vi "AuMT8852B Dirty Parameter Table.vi"(0 "VISA session":refnum<visa-resource-name>, 1 "Test (Single-slot sensitivity)":T1(ring), 2 "Variable (Frequency offset)":T2(ring), 3 "Range check? (F)":bool, 4 "Simulate? (F)":bool, 5 "error in (no error)":errorcluster, 6 "Set/Get (Set)":enum16{"Set", "Get"}(ring), 8 "Script (3)":i32=3, 10 "Parameters":dbl[](array[numeric]) format="%.2f") -> (13 "Parameters out":dbl[](array[numeric]) format="%.2f", 14 "VISA session out":refnum<visa-resource-name>, 19 "error out":errorcluster)   [LabVIEW 2017]
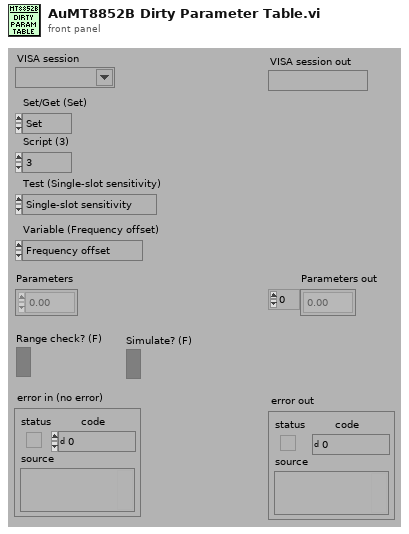
[diagram p1: front panel]
types:
  T1 = enum16{"Single-slot sensitivity", "Multiple-slot sensitivity", "EDR sensitivity"}
  T2 = enum16{"Frequency offset", "Symbol timing value", "Mod index value"}
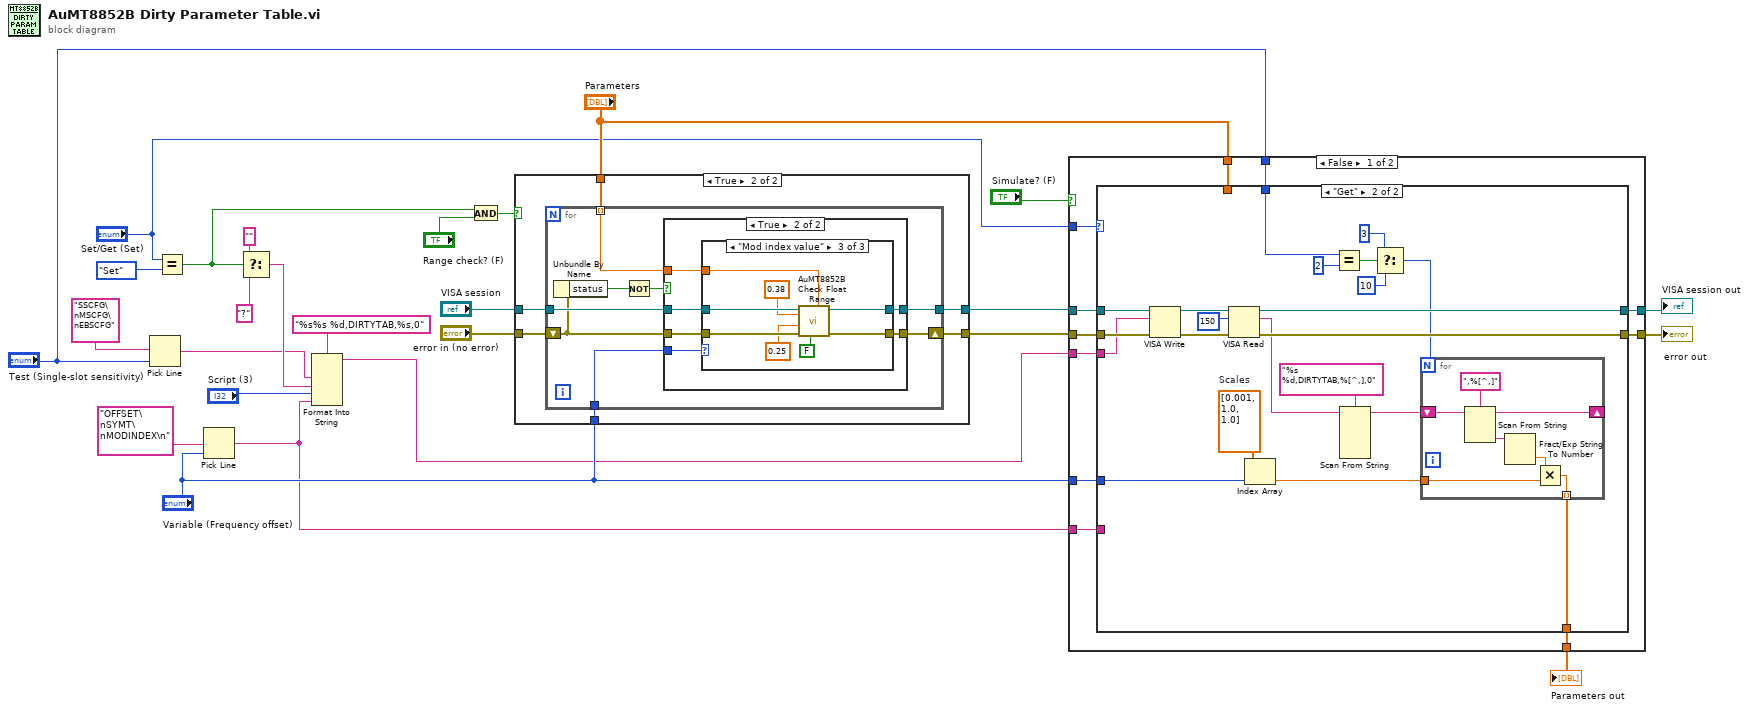
[diagram p0: block diagram]
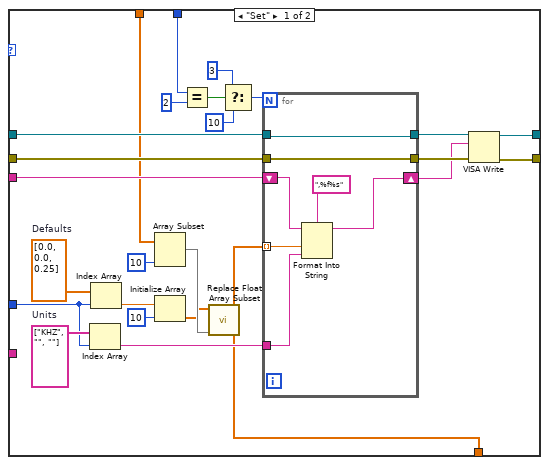
[diagram p2: hidden frame]
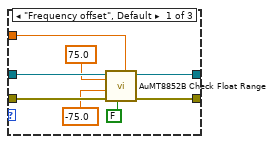
[diagram p6: hidden frame]
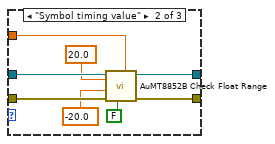
[diagram p7: hidden frame]
diagram:
  n1 = Pick Line(multi-line string="SSCFG\nMSCFG\nEBSCFG", line index="Test (Single-slot sensitivity)") -> (output string=w2:string)  [unwired: 1 in]
  n2 = Equal?(x="Set/Get (Set)", y=enum16{"Set", "Get"}."Set") -> (x = y?=w15:bool)
  n3 = Pick Line(multi-line string="OFFSET\nSYMT\nMODINDEX\n", line index="Variable (Frequency offset)") -> (output string=w5:string)  [unwired: 1 in]
  n4 = Select(t="", s=w15, f="?") -> (s? t:f=w21:string)
  n5 = Format Into String(format string="%s%s %d,DIRTYTAB,%s,0" ("Format String"), w2, w21, "Script (3)", w5) -> (resulting string=w6:string)  [unwired: 2 in, 1 out]
  n6 = And(x=w15, y="Range check? (F)") -> (x .and. y?=w17:bool)
  n7 = case shown="True" w17 {
    tunnel: "VISA session" -> [w28 w34]
    tunnel: "error in (no error)" -> [w27 w30]
    tunnel: [w28 w33] -> w13
    tunnel: [w27 w29] -> w14
    tunnel: "Parameters" -> [_ w32]
    tunnel: "Variable (Frequency offset)" -> [_ w31]
    frame False {
    }
    frame True {
      n8 = for {
        tunnel: w34 -> [w42]
        tunnel: [w41] -> w33
        tunnel: w32 -> [w39] mode=indexing
        tunnel: w31 -> [w40]
        shift-right: [w36] -> w29
        shift-left: w30 -> [w35]
        n9 = Unbundle By Name(w35) -> ("status"=w37:bool)
        n10 = Not(x=w37) -> (.not. x?=w38:bool)
        n11 = case shown="True" w38 {
          tunnel: w42 -> [w43 w50]
          tunnel: w35 -> [w44 w49]
          tunnel: [w43 w48] -> w41
          tunnel: [w44 w47] -> w36
          tunnel: w40 -> [_ w46]
          tunnel: w39 -> [_ w45]
          frame False {
          }
          frame True {
            n12 = case shown="\"Mod index value\"" w46 {
              tunnel: w50 -> [w58 w66 w74]
              tunnel: w49 -> [w57 w65 w73]
              tunnel: [w56 w64 w72] -> w48
              tunnel: [w55 w63 w71] -> w47
              tunnel: w45 -> [w51 w59 w67]
              frame "Frequency offset", Default {
                n13 = call <instrlib>:"AuMT8852B Check Float Range.vi"("Value (0)"=w51, "Check IVI flag first? (T)"=FALSE, "error in (no error)"=w57, "Lower limit (-1)"=-75.0, "Upper limit (1)"=75.0, "VISA session"=w58) -> ("error out"=w55:errorcluster, "VISA session out"=w56:refnum<visa-resource-name>)  [unwired: 4 in]
              }
              frame "Symbol timing value" {
                n14 = call <instrlib>:"AuMT8852B Check Float Range.vi"("Value (0)"=w59, "Check IVI flag first? (T)"=FALSE, "error in (no error)"=w65, "Lower limit (-1)"=-20.0, "Upper limit (1)"=20.0, "VISA session"=w66) -> ("error out"=w63:errorcluster, "VISA session out"=w64:refnum<visa-resource-name>)  [unwired: 4 in]
              }
              frame "Mod index value" {
                n15 = call <instrlib>:"AuMT8852B Check Float Range.vi"("Value (0)"=w67, "Check IVI flag first? (T)"=FALSE, "error in (no error)"=w73, "Lower limit (-1)"=0.25, "Upper limit (1)"=0.38, "VISA session"=w74) -> ("error out"=w71:errorcluster, "VISA session out"=w72:refnum<visa-resource-name>)  [unwired: 4 in]
              }
            }
          }
        }
      }
    }
  }
  n16 = case shown="False" "Simulate? (F)" {
    tunnel: w13 -> [w85 w148]
    tunnel: w14 -> [w84 w147]
    tunnel: [w83 w148] -> w12
    tunnel: [w82 w147] -> w11
    tunnel: [w81 w146] -> w4
    tunnel: "Parameters" -> [w79 w146]
    tunnel: "Set/Get (Set)" -> [w80 _]
    tunnel: "Variable (Frequency offset)" -> [w78 _]
    tunnel: w6 -> [w77 _]
    tunnel: w5 -> [w76 _]
    tunnel: "Test (Single-slot sensitivity)" -> [w75 _]
    frame False {
      n17 = case shown="\"Get\"" w80 {
        tunnel: w85 -> [w110 w138]
        tunnel: w84 -> [w109 w137]
        tunnel: [w104 w133] -> w83
        tunnel: [w106 w132] -> w82
        tunnel: [w94 w130] -> w81
        tunnel: w79 -> [w98 _]
        tunnel: w78 -> [w95 w124]
        tunnel: w77 -> [w108 w131]
        tunnel: w76 -> [_ _]
        tunnel: w75 -> [w86 w118]
        frame "Set" {
          w101 = string[] ["KHZ", "", ""]  # Units
          w102 = dbl[] [0.0, 0.0, 0.25]  # Defaults
          n18 = Index Array(array=w101, index=w95) -> (element=w96:string)
          n19 = Index Array(array=w102, index=w95) -> (element=w100:dbl)
          n20 = Array Subset(array=w98, length=10) -> (w93:dbl[])  [unwired: 1 in]
          n21 = Initialize Array(w100, 10 ("dimension size")) -> (w92:dbl[])
          n22 = Equal?(x=w86, y=2) -> (x = y?=w88:bool)
          n23 = call <instrlib>:"Replace Float Array Subset.vi"("New elements"=w93, "Input array"=w92) -> ("Output array"=w94:dbl[])  [unwired: 2 in]
          n24 = Select(t=3, s=w88, f=10) -> (s? t:f=w90:i32)
          n25 = for {
            N: w90 -> [_]
            tunnel: w110 -> [w114]
            tunnel: w109 -> [w115]
            tunnel: [w115] -> w107
            tunnel: [w114] -> w105
            shift-right: [w113] -> w103
            shift-left: w108 -> [w116]
            tunnel: w94 -> [w112] mode=indexing
            tunnel: w96 -> [w111]
            n26 = Format Into String(format string=",%f%s" ("Format String"), initial string=w116, w112, w111) -> (resulting string=w113:string)  [unwired: 1 in, 1 out]
          }
          n27 = VISA Write(VISA resource name=w105, write buffer=w103, error in (no error)=w107) -> (VISA resource name out=w104:refnum<visa-resource-name>, error out=w106:errorcluster)  [unwired: 1 out]
        }
        frame "Get" {
          w126 = dbl[] [0.001, 1.0, 1.0]  # Scales
          n28 = VISA Write(VISA resource name=w138, write buffer=w131, error in (no error)=w137) -> (VISA resource name out=w136:refnum<visa-resource-name>, error out=w135:errorcluster)  [unwired: 1 out]
          n29 = VISA Read(VISA resource name=w136, byte count=u32 150 ("byte count (0)"), error in (no error)=w135) -> (VISA resource name out=w133:refnum<visa-resource-name>, read buffer=w127:string, error out=w132:errorcluster)  [unwired: 1 out]
          n30 = Index Array(array=w126, index=w124) -> (element=w125:dbl)
          n31 = Equal?(x=w118, y=2) -> (x = y?=w121:bool)
          n32 = Scan From String(format string="%s %d,DIRTYTAB,%[^,],0", input string=w127) -> (remaining string=w128:string)  [unwired: 8 in, 2 out]
          n33 = Select(t=3, s=w121, f=10) -> (s? t:f=w119:i32)
          n34 = for {
            N: w119 -> [_]
            shift-right: [w144] -> _
            shift-left: w128 -> [w145]
            tunnel: [w140] -> w130 mode=indexing
            tunnel: w125 -> [w139]
            n35 = Scan From String(format string=",%[^,]", input string=w145) -> (remaining string=w144:string, output 1=w142:string)  [unwired: 3 in, 2 out]
            n36 = Fract/Exp String To Number(string=w142) -> (number=w141:dbl)  [unwired: 3 in, 1 out]
            n37 = Multiply(x=w141, y=w139) -> (x*y=w140:dbl)
          }
        }
      }
    }
    frame True {
    }
  }
  "VISA session out" <- w12
  "error out" <- w11
  "Parameters out" <- w4
